vi "DSF.Engine.Runtime.Framework.Shutdown.vi"(8 "error in (no error)":errorcluster, 11 "Framework Runtime in":refnum<class "DSF.Engine.Runtime.Framework.lvclass">) -> (0 "error out":errorcluster, 3 "Framework Runtime out":refnum<class "DSF.Engine.Runtime.Framework.lvclass">)   [LabVIEW 2016, in "DSF.Engine.lvlib" / "DSF.Engine.Runtime.Framework.lvclass"]
uses:
  DSF.Engine.Runtime.Framework.lvclass
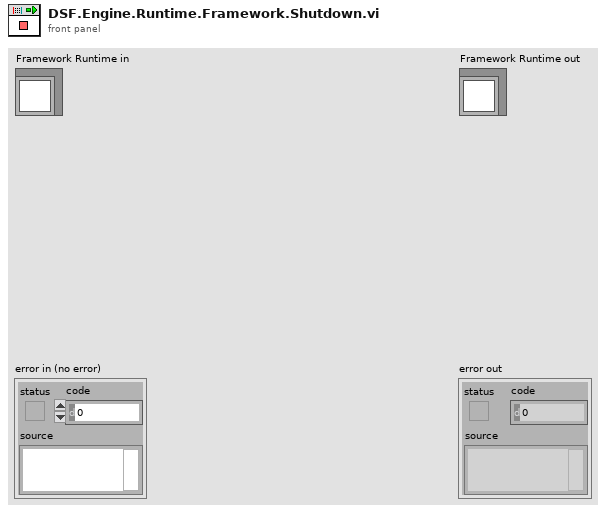
[diagram p1: front panel]
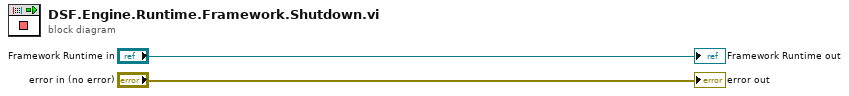
[diagram p0: block diagram]
diagram:
  "error out" <- "error in (no error)"
  "Framework Runtime out" <- "Framework Runtime in"
